vi "Set Active Tag.vi"(8 "error in (no error)":errorcluster, 11 "Tag_LVOOP in":refnum<class "Tree Tag Class.lvclass">) -> (0 "error out":errorcluster, 3 "Tag_LVOOP out":refnum<class "Tree Tag Class.lvclass">)   [LabVIEW 2012, in "Tree Tools.lvlib" / "Tree Tag Class.lvclass"]
uses:
  Tree Tag Class.lvclass
  Tree Tag Class.lvclass/Tree Tag Class.ctl
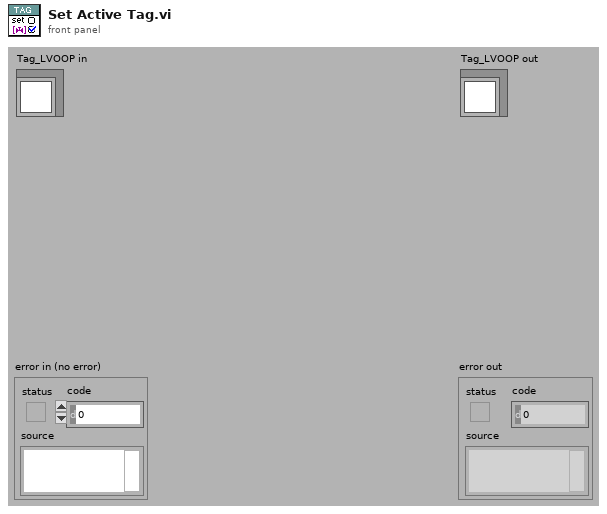
[diagram p1: front panel]
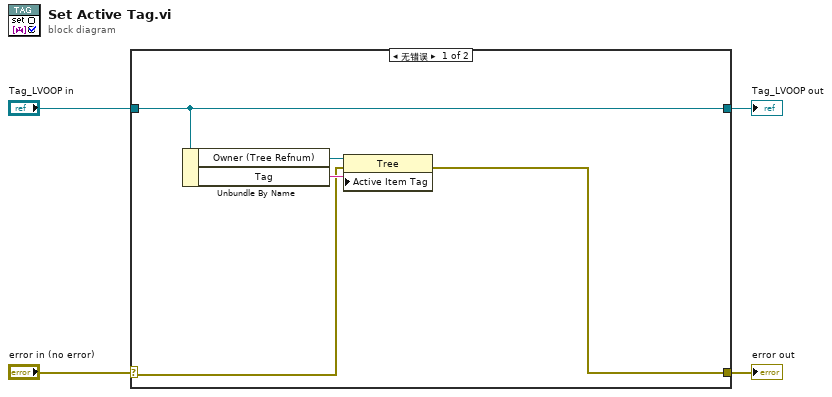
[diagram p0: block diagram]
diagram:
  n1 = case shown="无错误" "error in (no error)" {
    selector: "error in (no error)" -> [w5 w11]
    tunnel: [w6 w11] -> w3
    tunnel: [w9 w10] -> w1
    tunnel: "Tag_LVOOP in" -> [w9 w10]
    frame No Error {
      n2 = Unbundle By Name(w9) -> ("Owner (Tree Refnum)"=w8:refnum<vi>, "Tag"=w7:string)
      n3 = property class="Tree"(reference=w8, error in=w5, "Active Item Tag"=w7) -> (error out=w6:errorcluster)  [unwired: 1 out]
    }
    frame Error {
    }
  }
  "error out" <- w3
  "Tag_LVOOP out" <- w1
